vi "Teleop.vi"(10 "Match Info":T1={"Autonomous Elapsed Seconds"=0.0, "TeleOp Elapsed Seconds"=0.0, "Disabled Elapsed Seconds"=0.0, "Visited Autonomous"=FALSE, "Visited TeleOp"=FALSE, "Visited Disabled"=FALSE, "Autonomous Settings"={"Autonomous Style"=enum."Independent", "VI Refnum"=refnum}}, 11 "Call Context":T2) -> ()   [LabVIEW 2017]
doc: "This VI is called for each TeleOp packet received from the DS where the robot is not disabled. It is often used to read from the joysticks and update I/O or to update setpoints for timed control loops. It should complete and return within 20 milliseconds or it may miss DS packets."
uses:
  <vilib>/Rock Robotics/WPI/DriverStation/WPI_DriverStationDerivedRobotMode.ctl
  <vilib>/Rock Robotics/WPI/DriverStation/WPI_DriverStationMatch Info.ctl
  _SOURCE2018_Master/_SHARE ALL/TypeDef Share All/ENUM_Joystick_Buttons.ctl
  _SOURCE2018_Master/_SHARE ALL/TypeDef Share All/ENUM_Joystick_Axes.ctl
  _SOURCE2018_Master/_SHARE ALL/RoboRio Share All/SRX Share All/TypeDefs SRX/Cluster_SRX_Mode and Value.ctl
  _SOURCE2018_Master/System Drivers/Phoenix-LabVIEW/Motor Controller/Controls/CTRE_Phoenix_MotorControl_ControlMode.ctl
  _SOURCE2018_Master/_SHARE ALL/RoboRio Share All/Systems Share All/Joystick/Global_Joystick Write_Data.vi
  Globals/CMD_Global.vi
  _SOURCE2018_Master/_SHARE ALL/RoboRio Share All/Systems Share All/Joystick/Joystick.lvlib
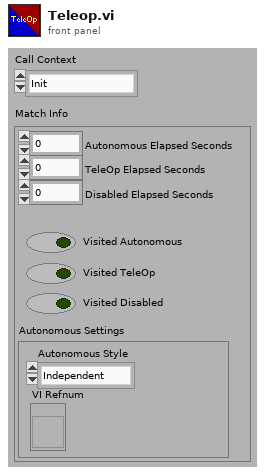
[diagram p1: front panel]
types:
  T1 = typedef "WPI_DriverStationMatch Info.ctl" = cluster{"Autonomous Elapsed Seconds":dbl, "TeleOp Elapsed Seconds":dbl, "Disabled Elapsed Seconds":dbl, "Visited Autonomous":bool, "Visited TeleOp":bool, "Visited Disabled":bool, "Autonomous Settings":cluster{"Autonomous Style":enum16{"Iterative", "Independent"}, "VI Refnum":refnum<vi>}}
  T2 = typedef "WPI_DriverStationDerivedRobotMode.ctl" = enum16{"Init", "Execute", "Stop"}
  T3 = typedef "CTRE_Phoenix_MotorControl_ControlMode.ctl" = u16
  T4 = typedef "Cluster_SRX_Mode and Value.ctl" = cluster{"Mode":T3, "Value":dbl}
  T5 = typedef "ENUM_Joystick_Axes.ctl" = enum16{"Left X", "Left Y", "Left Trigger", "Right Trigger", "Right X", "Right Y"}
  T6 = typedef "ENUM_Joystick_Buttons.ctl" = enum16{"Green A", "Red B", "Blue X", "Yellow Y", "Left Bumper", "Right Bumper", "Back", "Start", "Left Joystick", "Right Joystick"}
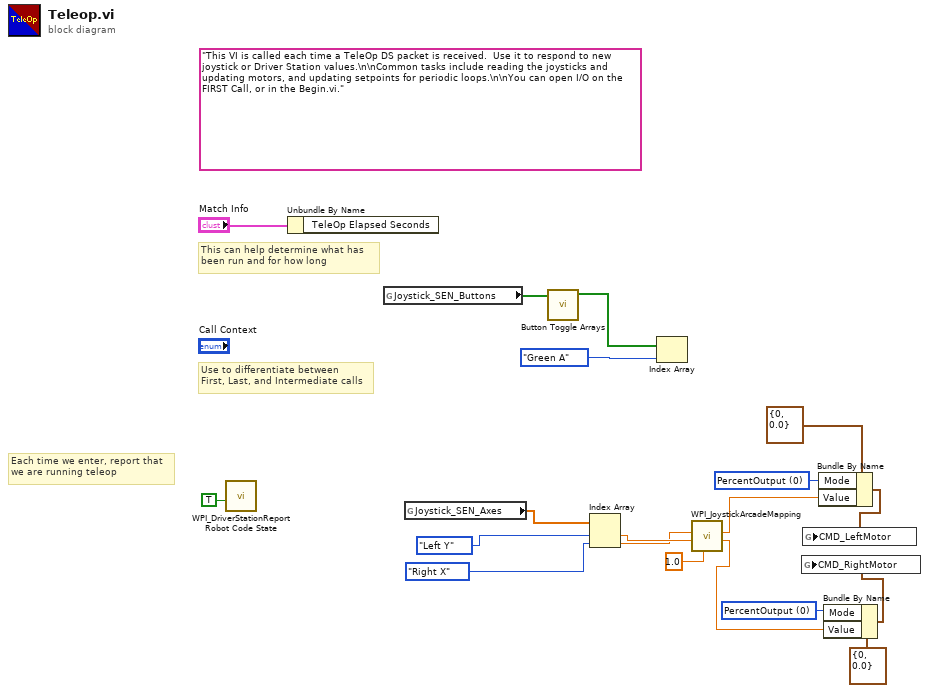
[diagram p0: block diagram]
diagram:
  w3 = T3 0 items=["PercentOutput"=0, "Position"=1, "Velocity"=2, "Current"=3, "Follower"=5, "MotionProfile"=6, "MotionMagic"=7, "MotionMagicArc"=8, "MotionProfileArc"=10, "Disabled"=15] ("Mode")
  w7 = T3 0 items=["PercentOutput"=0, "Position"=1, "Velocity"=2, "Current"=3, "Follower"=5, "MotionProfile"=6, "MotionMagic"=7, "MotionMagicArc"=8, "MotionProfileArc"=10, "Disabled"=15] ("Mode")
  (unwired) "This VI is called each time a TeleOp DS packet is received.  Use it to respond to new joystick or Driver Station values.\n\nCommon tasks include reading the joysticks and updating motors, and updating setpoints for periodic loops.\n\nYou can open I/O on the FIRST Call, or in the Begin.vi."
  # "Each time we enter, report that\nwe are running teleop"
  # "Use to differentiate between\nFirst, Last, and Intermediate calls"
  # "This can help determine what has\nbeen run and for how long"
  n1 = call <vilib>:"WPI_DriverStationReport Robot Code State.vi"("TeleOp"=TRUE ("Autonomous")) -> ()  [unwired: 10 in, 1 out]
  n2 = Unbundle By Name("Match Info") -> ()  [unwired: 1 out]
  n3 = global read "Global_Joystick Write_Data.vi" "Joystick_SEN_Buttons"() -> (w16:bool[])
  n4 = global read "Global_Joystick Write_Data.vi" "Joystick_SEN_Axes"() -> (w14:dbl[])
  n5 = call "Button Toggle Arrays.vi"("Joystick_SEN_Buttons"=w16) -> ("Toggle Outputs Out"=w15:bool[])  [unwired: 8 in, 2 out]
  n6 = Index Array(array=w14, index #1=ENUM_Joystick_Axes."Left Y" ("index"), index #2=ENUM_Joystick_Axes."Right X" ("index")) -> (element #1=w11:dbl, element #2=w10:dbl)
  n7 = Index Array(array=w15, index=ENUM_Joystick_Buttons."Green A") -> ()  [unwired: 1 out]
  n8 = call <vilib>:"WPI_JoystickArcadeMapping.vi"("Max Output"=1.0, "Y axis value"=w11, "X axis value"=w10) -> ("Right Motor Value"=w1:dbl, "Left Motor Value"=w2:dbl)  [unwired: 7 in]
  n9 = Bundle By Name(cluster=T4 {"Mode"=0, "Value"=0.0} ("Mode And Value"), "Mode"=w7, "Value"=w2) -> (w6:T4)
  n10 = global write "CMD_Global.vi" "CMD_LeftMotor"(w6) -> ()
  n11 = Bundle By Name(cluster=T4 {"Mode"=0, "Value"=0.0} ("Mode And Value"), "Mode"=w3, "Value"=w1) -> (w4:T4)
  n12 = global write "CMD_Global.vi" "CMD_RightMotor"(w4) -> ()
